vi "filterWheelMove.vi"(1 "filter index":u8(ring) items=["ch_BFP", "ch_Cerulean", "ch_GFP", "ch_mOrange", "ch_mCherry", "ch_mNeptune"]) -> (0 "read buffer":string)   [LabVIEW 2017]
uses:
  globalDevices.vi
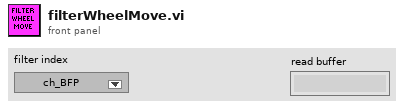
[diagram p1: front panel]
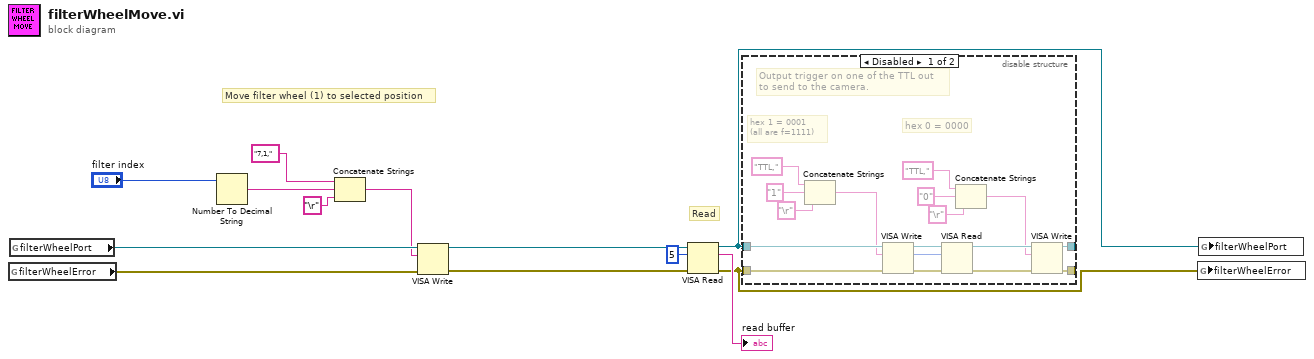
[diagram p0: block diagram]
diagram:
  # "Read"
  # "Move filter wheel (1) to selected position"
  n1 = global read "globalDevices.vi" "filterWheelError"() -> (w12:errorcluster)
  n2 = global read "globalDevices.vi" "filterWheelPort"() -> (w13:refnum<visa-resource-name>)
  n3 = Number To Decimal String(number="filter index") -> (decimal integer string=w10:string)  [unwired: 1 in]
  n4 = Concatenate Strings("7,1,", w10, "\r" ("string")) -> (w9:string)
  n5 = VISA Write(VISA resource name=w13, write buffer=w9, error in (no error)=w12) -> (VISA resource name out=w7:refnum<visa-resource-name>, error out=w6:errorcluster)  [unwired: 1 out]
  n6 = VISA Read(VISA resource name=w7, byte count=u32 5, error in (no error)=w6) -> (VISA resource name out=w2:refnum<visa-resource-name>, read buffer=→"read buffer":string, error out=w3:errorcluster)  [unwired: 1 out]
  n7 = disable-structure shown="Disabled" {
    disable-tunnel: w2 -> [w28 _]
    disable-tunnel: w3 -> [w27 _]
    disable-tunnel: [w17 _] -> _
    disable-tunnel: [w16 _] -> _
    frame Disabled {
      # "hex 0 = 0000"
      # "hex 1 = 0001\n(all are f=1111)"
      # "Output trigger on one of the TTL out\nto send to the camera."
      n8 = Concatenate Strings("TTL," ("string"), "1" ("string"), "\r" ("string")) -> (w26:string)
      n9 = VISA Write(VISA resource name=w28, write buffer=w26, error in (no error)=w27) -> (VISA resource name out=w23:refnum<visa-resource-name>, return count=w24:u32, error out=w25:errorcluster)
      n10 = VISA Read(VISA resource name=w23, byte count=w24, error in (no error)=w25) -> (VISA resource name out=w22:refnum<visa-resource-name>, error out=w21:errorcluster)  [unwired: 2 out]
      n11 = Concatenate Strings("TTL," ("string"), "0" ("string"), "\r" ("string")) -> (w18:string)
      n12 = VISA Write(VISA resource name=w22, write buffer=w18, error in (no error)=w21) -> (VISA resource name out=w17:refnum<visa-resource-name>, error out=w16:errorcluster)  [unwired: 1 out]
    }
    frame Enabled {
    }
  }
  n13 = global write "globalDevices.vi" "filterWheelError"(w3) -> ()
  n14 = global write "globalDevices.vi" "filterWheelPort"(w2) -> ()
